vi "Index volume data.vi"(9 "Cycle index":i32, 10 "Single trial data (single channel)":u16[](array[numeric]), 11 "Parameters Cluster":T1) -> (0 "<Points in all volumes/trials>":i32, 3 "3D":u16[][][](array[numeric]), 4 "Points in each cycle":i32, 6 "Points in each cycle (fractional)":dbl)   [LabVIEW 2020]
panel:
  out "size(s)":i32[](array[numeric])
  # "Re-entrant"
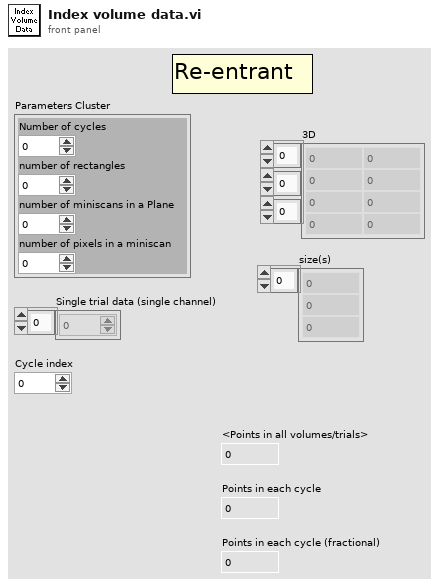
[diagram p1: front panel]
types:
  T1 = cluster{"Number of cycles":i32, "number of rectangles":i32, "number of miniscans in a Plane":i32, "number of pixels in a miniscan":i32}
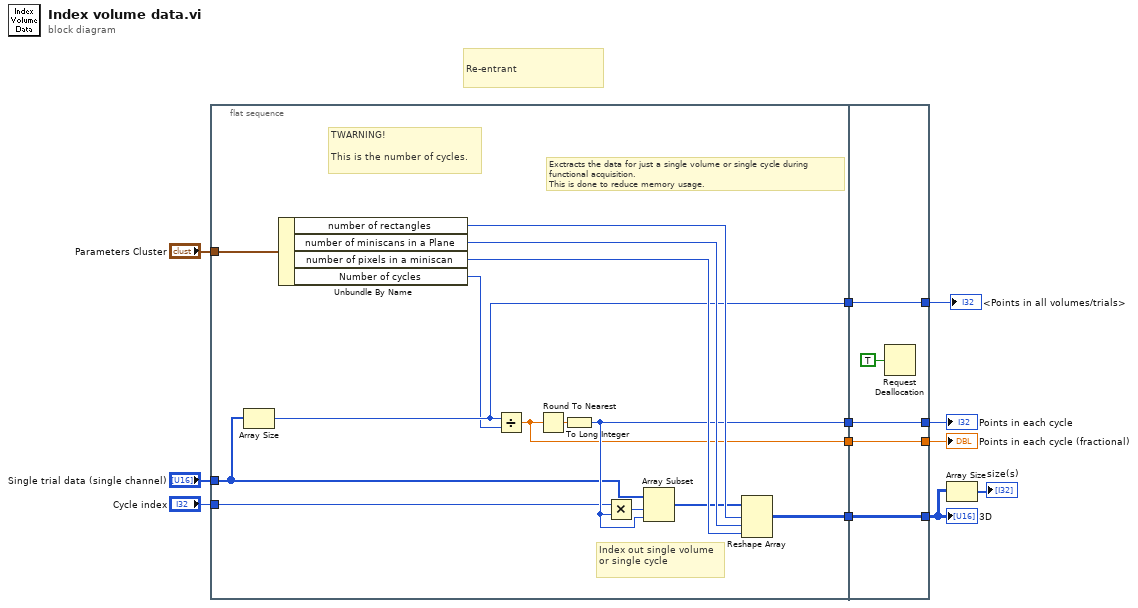
[diagram p0: block diagram]
diagram:
  # "Re-entrant"
  n1 = flat-sequence {
    tunnel: "Cycle index" -> [w19]
    tunnel: "Parameters Cluster" -> [w16]
    tunnel: "Single trial data (single channel)" -> [w14]
    tunnel: [w26] -> w6
    tunnel: [w21] -> w5
    tunnel: [w20] -> w4
    tunnel: [w17] -> w3
    tunnel: [w28] -> w9
    tunnel: [w29] -> w11
    tunnel: [w30] -> w12
    tunnel: [w31] -> w2
    tunnel: w6 -> [w31]
    tunnel: w5 -> [w30]
    tunnel: w4 -> [w29]
    tunnel: w3 -> [w28]
    frame #0 {
      # "Exctracts the data for just a single volume or single cycle during functional acquisition.\nThis is done to reduce memory usage."
      # "TWARNING!\n\nThis is the number of cycles."
      # "Index out single volume or single cycle"
      n2 = Array Size(array=w14) -> (size(s)=w20:i32)
      n3 = Unbundle By Name(w16) -> ("number of rectangles"=w23:i32, "number of miniscans in a Plane"=w24:i32, "number of pixels in a miniscan"=w25:i32, "Number of cycles"=w13:i32)
      n4 = Divide(x=w20, y=w13) -> (x/y=w17:dbl)
      n5 = Round To Nearest(number=w17) -> (nearest integer value=w15:dbl)
      n6 = To Long Integer(number=w15) -> (32bit integer=w21:i32)
      n7 = Multiply(x=w19, y=w21) -> (x*y=w18:i32)
      n8 = Array Subset "Array Subset"(array=w14, index=w18, length=w21) -> (w22:u16[])
      n9 = Reshape Array(w22, w23, w24, w25) -> (w26:u16[][][])
    }
    frame #1 {
      n10 = Request Deallocation(TRUE ("flag")) -> ()
    }
  }
  n11 = Array Size(array=w2) -> (size(s)=→"size(s)":i32[])
  "3D" <- w2
  "Points in each cycle" <- w12
  "<Points in all volumes/trials>" <- w11
  "Points in each cycle (fractional)" <- w9
